vi "Configure Delimiter.vi"(8 "Error In":errorcluster, 11 "Delimiter":string=",") -> (0 "Error Out":errorcluster)   [LabVIEW 2018, in "Toolkit.lvlib"]
doc: "Changes the default delimiter for columns, or fields, in each line, or record, of the log file. The default is the comma."
uses:
  Toolkit.lvlib
  Support/File/Action.ctl
  Support/File/File.lvlib
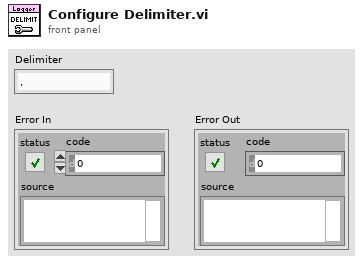
[diagram p1: front panel]
types:
  T1 = typedef "Toolkit.lvlib/File.lvlib/Action.ctl" = enum16{"Initialize", "Set Maximum File Size", "Set Maximum File Count", "Set Root Folder", "Set Enable Calendar Folder Tree", "Set File Extension", "Set Prune All", "Set Delimiter", "Start", "Write", "Stop", "Shutdown"}
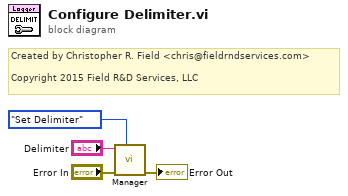
[diagram p0: block diagram]
diagram:
  # "Created by Christopher R. Field <chris@fieldrndservices.com>\n\nCopyright 2015 Field R&D Services, LLC"
  n1 = call "Manager.vi"("Action"=Action."Set Delimiter", "Error In"="Error In", "Set Value"="Delimiter") -> ("Error Out"=→"Error Out":errorcluster)  [unwired: 8 in]
